vi "SDI-12 Continuous Operations.vi"(0 "RS232 Port In":refnum<visa-resource-name>="COM11", 1 "Sensor Address In":string="0", 3 "Sonde Data Ctl Refnum":refnum<vi>, 4 "Stop Ctl Refnum":refnum<vi>, 5 "Error In (No Error)":errorcluster, 6 "file directory (dialog if empty)":path=path "D:/Cascade/Raw Data files", 7 "Save File":bool) -> (11 "Measurements Out":dbl[](array[numeric]), 12 "new file path (Not A Path if cancelled)":path, 13 "Array":timestamp[](array[timestamp]), 15 "Address Out":string="a" caption="sensor address out", 16 "output cluster":T1 caption="Cluster" {"Dissolved\nOxygen %" format="%_4g"; "Salinity" format="%_3g"; "Temp deg C" format="%_2g"; "ORP" format="%_4g"; "pH" format="%_4g"; "Dissolved\nOxygen mg/L" format="%_4g"; "Specific\nCond (uS)" format="%_4g"}, 17 "Temperature":cluster{"Y":dbl[], "Y":dbl[]}[](graph), 18 "Sonde Data Display":T2, 19 "Error Out":errorcluster)   [LabVIEW 2016]
doc: "A general set of examples of the SDI-12 API for a generic sensor. A tab control separates each example, and contains the following examples:\n1. Read Single.\n2. Read Multiple.\n3. Acknowledge Active.\n4. Change Address.\n5. Address Query.\n6. Send Identification."
uses:
  SDI-12/Sonde Vertical Graph.ctl
  controls/Vertical Chart.ctl
  activeXtest/activeXtest 2015 Folder/sonde cluster.ctl
  <vilib>/Utility/file.llb/Write Delimited Spreadsheet (string).vi
  <vilib>/Utility/file.llb/Write Delimited Spreadsheet (DBL).vi
  SDI-12/SDI-12.lvlib
panel:
  out "Sensor On/Off Response":bool
  out "Battery Voltage (V)":dbl
  out "Number of Measurements Out":i32
  in  "Measurement Type In (Normal)":i32(ring)=1 items=["Normal", "Concurrent", "Continuous"]
  out "Parameter Out":i32(ring) items=["0", "1", "2", "3", "4", "5", "6", "7", "8", "9"]
  in  "Parameter In (0)":i32(ring) items=["0", "1", "2", "3", "4", "5", "6", "7", "8", "9"]
  in  "CRC (False)":bool
  out "CRC Out":bool
  out "Measurement Type Out":i32(ring) items=["Normal", "Concurrent", "Continuous"]
  out "Time (s)":dbl
  in  "stop":bool
  out "counter":i32
  out "start time":timestamp
  # "deg C"
  # "pH"
  # "specific conductance"
  # "salinity"
  # "DO % saturation"
  # "DO mg/L"
  # "ORP"
  # "depth"
  # "battery"
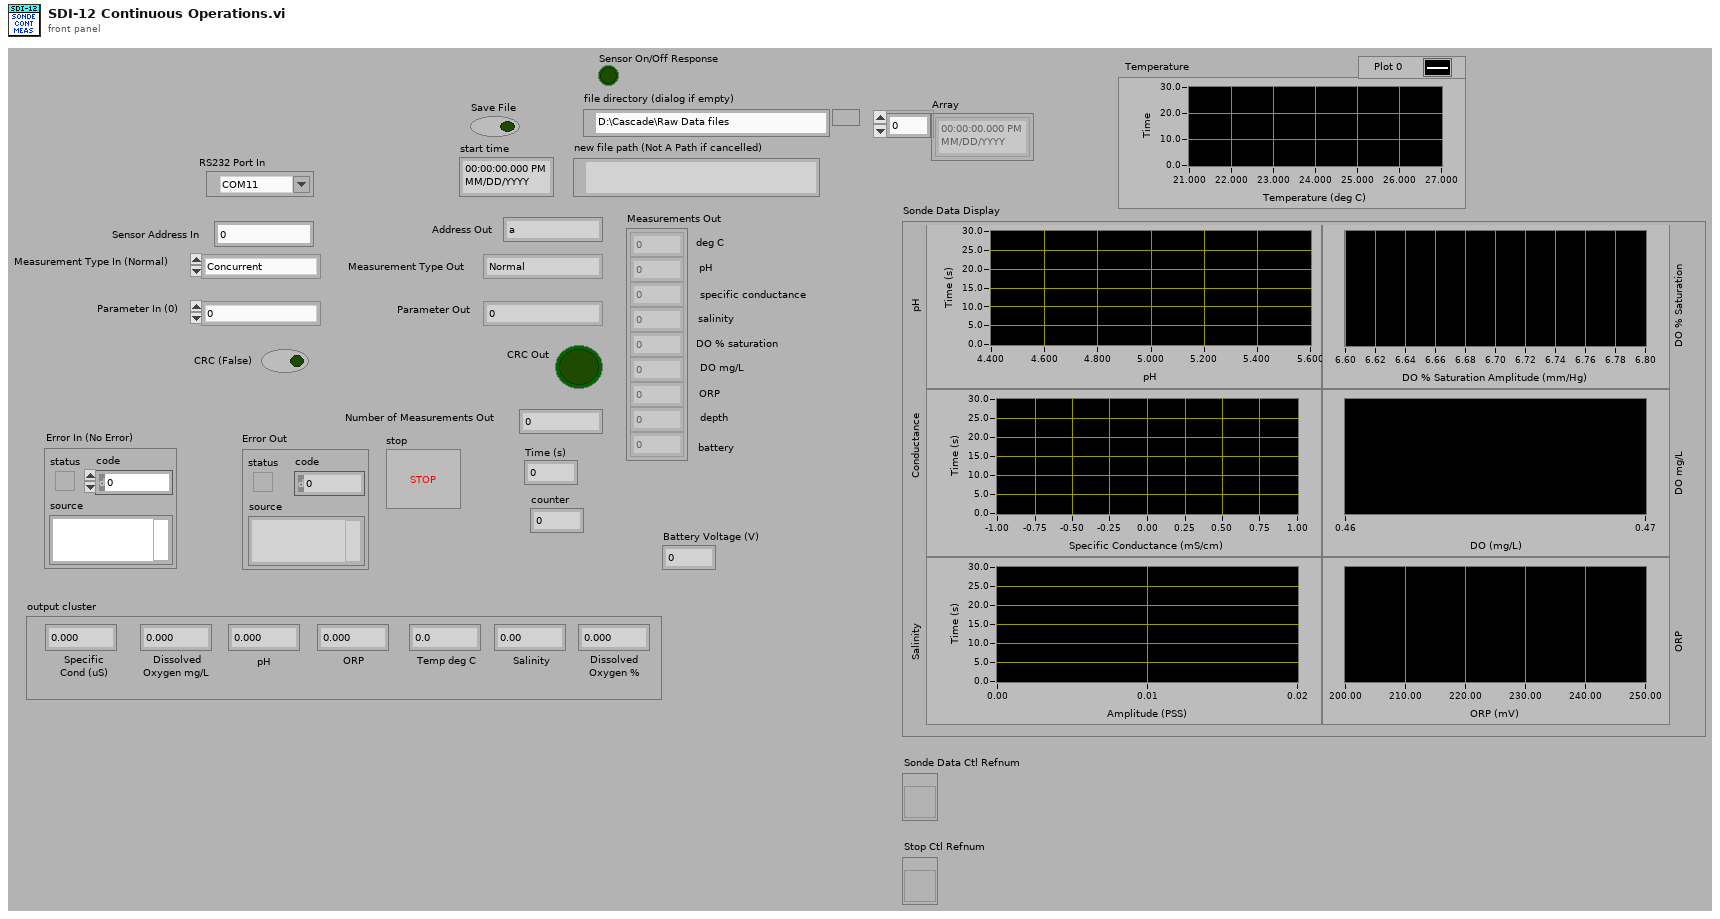
[diagram p1: front panel]
types:
  T1 = typedef "sonde cluster.ctl" = cluster{"Specific\nCond (uS)":dbl, "Dissolved\nOxygen mg/L":dbl, "pH":dbl, "ORP":dbl, "Temp deg C":dbl, "Salinity":dbl, "Dissolved\nOxygen %":dbl}
  T2 = typedef "Sonde Vertical Graph.ctl" = cluster{"pH":T3, "Conductance":T3, "Salinity":T3, "DO % Saturation":T3, "DO mg/L":T3, "ORP":T3}
  T3 = typedef "Vertical Chart.ctl" = cluster{"Y":dbl[], "Y":dbl[]}[]
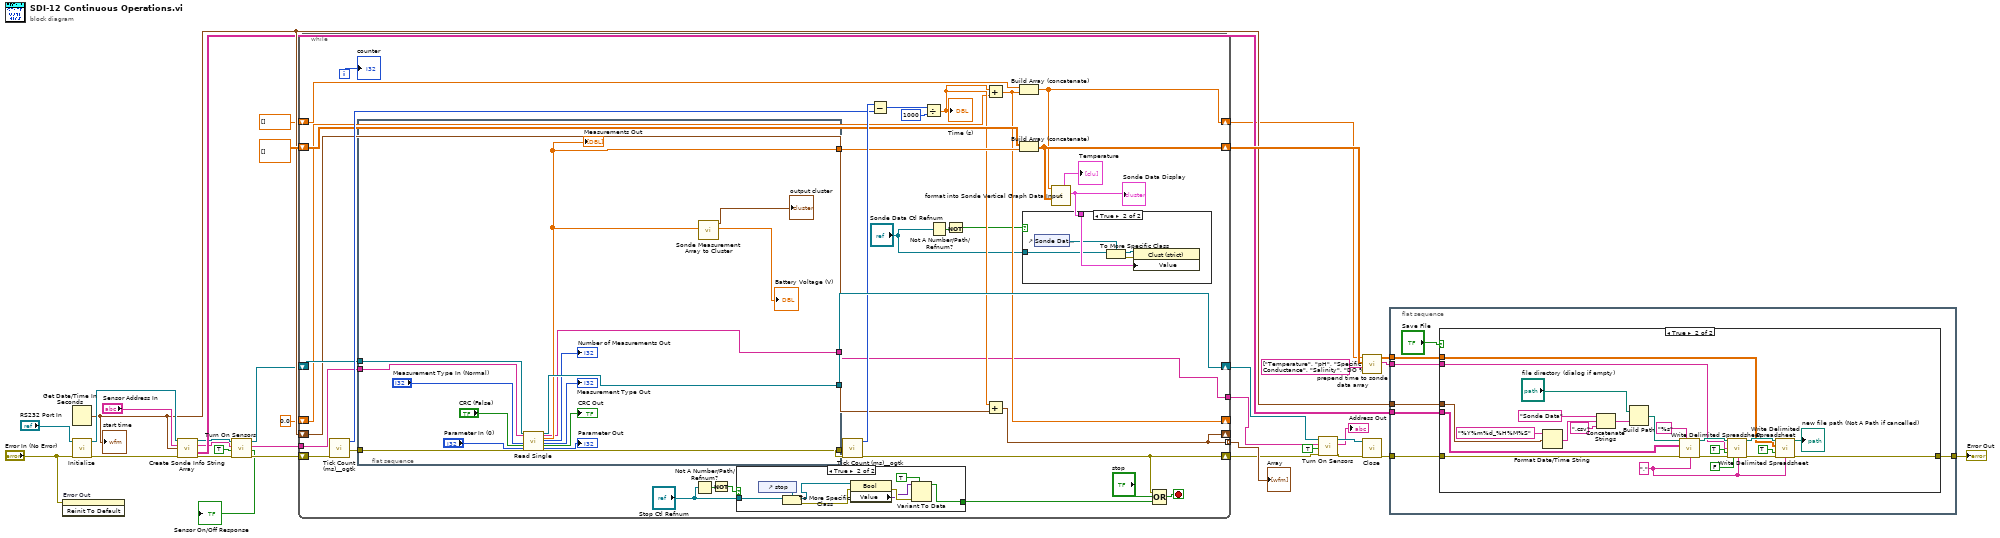
[diagram p0: block diagram]
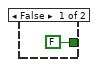
[diagram p3: hidden frame]
diagram:
  n1 = invoke on="Error Out" class="Clust (strict)" method="Reinit To Default"(error in="Error In (No Error)") -> ()  [unwired: 2 in, 3 out]
  n2 = Get Date/Time In Seconds() -> (seconds since 1Jan1904=w23:timestamp)
  "start time" <- w23
  n3 = call "Initialize.vi"("Error In (No Error)"="Error In (No Error)", "RS232 Port In"="RS232 Port In") -> ("Error Out"=w32:errorcluster, "RS232 Port Out"=w31:refnum<visa-resource-name>)  [unwired: 8 in]
  n4 = call "Create Sonde Info String Array.vi"("VISA Refnum in"=w31, "Sensor Address In"="Sensor Address In", "seconds since 1Jan1904"=w23, "error in (no error)"=w32) -> ("VISA Refnum out"=w14:refnum<visa-resource-name>, "Address Out"=w12:string, "Array"=w22:string[][], "error out"=w16:errorcluster)  [unwired: 8 in]
  n5 = call "Turn On Sensors.vi"("Error In (No Error)"=w16, "Sensor On/Off"=TRUE, "Sensor Address In"=w12, "RS232 Port In"=w14) -> ("Error Out"=w15:errorcluster, "Sensor On/Off Response"=→"Sensor On/Off Response":bool, "Address Out"=w11:string, "RS232 Port Out"=w13:refnum<visa-resource-name>)  [unwired: 4 in]
  n6 = while {
    shift-right: [w67] -> w7
    shift-left: w13 -> [w60]
    shift-right: [w43] -> w9
    shift-left: w15 -> [w59]
    shift-right: [w54] -> w28
    shift-left: dbl[][] [] -> [w55]
    tunnel: [w52] -> w29 mode=indexing
    shift-right: [w52] -> _
    shift-left: w23 -> [w53]
    shift-right: [w50] -> w19
    shift-left: dbl[] [] -> [w47]
    tunnel: w11 -> [w51]
    shift-right: [w46] -> _
    shift-left: 0.0 -> [w48]
    tunnel: [w42] -> w5
    i -> [w57]
    stop <- w44 stop-if-true
    n7 = call <userlib>:"Tick Count (ms)__ogtk.vi"("error in (no error)"=w59) -> ("error out"=w65:errorcluster, "millisecond timer value"=w63:u32)  [unwired: 9 in]
    n8 = flat-sequence {
      tunnel: [w97] -> w67
      tunnel: [w96] -> w66
      tunnel: w65 -> [w88]
      tunnel: w60 -> [w87]
      tunnel: [w85] -> w56
      tunnel: w51 -> [w86]
      tunnel: [w84] -> w42
      frame #0 {
        n9 = call "Read Single.vi"("RS232 Port In"=w87, "Sensor Address In"=w86, "Measurement Type In (Normal)"="Measurement Type In (Normal)", "CRC (False)"="CRC (False)", "Parameter In (0)"="Parameter In (0)", "Error In (No Error)"=w88) -> ("RS232 Port Out"=w97:refnum<visa-resource-name>, "Sensor Address Out"=w84:string, "Measurements Out"=w85:dbl[], "Number of Measurements Out"=→"Number of Measurements Out":i32, "Measurement Type Out"=→"Measurement Type Out":i32, "CRC Out"=→"CRC Out":bool, "Parameter Out"=→"Parameter Out":i32, "Error Out"=w96:errorcluster)  [unwired: 14 in]
        "Measurements Out" <- w85
        n10 = call "Sonde Measurement Array to Cluster.vi"("Measurements In"=w85) -> ("Battery Voltage (V)"=→"Battery Voltage (V)":dbl, "Cluster Out"=→"output cluster":T1)  [unwired: 9 in]
      }
    }
    n11 = Not A Number/Path/Refnum?(number/path/refnum="Stop Ctl Refnum") -> (NaN/Path/Refnum?=w37:bool)
    n12 = Not(x=w37) -> (.not. x?=w35:bool)
    n13 = case shown="True" w35 {
      tunnel: "Stop Ctl Refnum" -> [_ w76]
      tunnel: [FALSE w69] -> w34
      frame False {
      }
      frame True {
        n14 = control-ref of="stop"() -> (w74:refnum<vi>)
        n15 = To More Specific Class(target class=w74, reference=w76) -> (specific class reference=w71:refnum<vi>, error out=w75:errorcluster)  [unwired: 1 in]
        n16 = property class="Bool"(reference=w71, error in=w75) -> (error out=w73:errorcluster, "Value"=w72:variant)  [unwired: 1 out]
        n17 = Variant To Data(error in=w73, type=TRUE, Variant=w72) -> (data=w69:bool)  [unwired: 1 out]
      }
    }
    n18 = call <userlib>:"Tick Count (ms)__ogtk.vi"("error in (no error)"=w66) -> ("error out"=w43:errorcluster, "millisecond timer value"=w64:u32)  [unwired: 9 in]
    n19 = Subtract(x=w64, y=w63) -> (x-y=w62:u32)
    n20 = Divide(x=w62, y=u32 1000) -> (x/y=w49:dbl)
    "Time (s)" <- w49
    n21 = Not A Number/Path/Refnum?(number/path/refnum="Sonde Data Ctl Refnum") -> (NaN/Path/Refnum?=w41:bool)
    n22 = Not(x=w41) -> (.not. x?=w40:bool)
    n23 = Add(x=w49, y=w48) -> (x+y=w46:dbl)
    n24 = Add(x=w49, y=w53) -> (x+y=w52:timestamp)
    n25 = Build Array (concatenate)(w47, w46) -> (w50:dbl[])
    n26 = Build Array (concatenate)(w55, w56) -> (w54:dbl[][])
    n27 = call "format into Sonde Vertical Graph Data Input.vi"("Sonde Measurement Array"=w54, "Time Array"=w50) -> ("Sonde Data Display"=w39:T2, "Temperature"=→"Temperature":cluster{"X":dbl[], "Y":dbl[]}[])  [unwired: 8 in]
    "Sonde Data Display" <- w39
    n28 = case shown="True" w40 {
      tunnel: w39 -> [_ w81]
      tunnel: "Sonde Data Ctl Refnum" -> [_ w79]
      frame False {
      }
      frame True {
        n29 = control-ref of="Sonde Data Display"() -> (w80:refnum<vi>)
        n30 = To More Specific Class(target class=w80, reference=w79) -> (specific class reference=w78:refnum<vi>, error out=w77:errorcluster)  [unwired: 1 in]
        n31 = property class="Clust (strict)"(reference=w78, error in=w77, "Value"=w81) -> ()  [unwired: 2 out]
      }
    }
    n32 = Compound Arithmetic op=OR(w43, "stop", w34) -> (w44:bool)
    "counter" <- w57
  }
  "Array" <- w29
  n33 = call "Turn On Sensors.vi"("Error In (No Error)"=w9, "Sensor On/Off"=TRUE, "Sensor Address In"=w5, "RS232 Port In"=w7) -> ("Error Out"=w8:errorcluster, "Address Out"=→"Address Out":string, "RS232 Port Out"=w6:refnum<visa-resource-name>)  [unwired: 4 in, 1 out]
  n34 = call "prepend time to sonde data array.vi"("Measurement Labels"=string[] ["Temperature", "pH", "Specific Conductance", "Salinity", "DO % saturation", "DO", "ORP", "depth", "battery"], "Sonde\nData Array"=w28, "Time Array"=w19) -> ("Header Array"=w21:string[], "Data Array"=w25:dbl[][])  [unwired: 7 in]
  n35 = call "Close.vi"("Error In (No Error)"=w8, "RS232 Port In"=w6) -> ("Error Out"=w27:errorcluster)  [unwired: 9 in]
  n36 = flat-sequence {
    tunnel: w27 -> [w104]
    tunnel: [w103] -> w26
    tunnel: w21 -> [w101]
    tunnel: w25 -> [w100]
    tunnel: w23 -> [w99]
    tunnel: w22 -> [w98]
    frame #0 {
      n37 = case shown="True" "Save File" {
        tunnel: [w105 w125] -> w103
        tunnel: w104 -> [w105 w110]
        tunnel: w101 -> [_ w106]
        tunnel: w100 -> [_ w123]
        tunnel: w99 -> [_ w117]
        tunnel: w98 -> [_ w108]
        frame False {
        }
        frame True {
          w107 = "," ("delimiter (\\t)")
          n38 = Format Date/Time String(time format string (%c)="%Y%m%d_%H%M%S", seconds (now)=w117) -> (date/time string=w116:string)  [unwired: 1 in]
          n39 = Concatenate Strings("Sonde Data" ("name or relative path"), w116, ".csv" ("string")) -> (w118:string)
          n40 = Build Path(base path="file directory (dialog if empty)", name or relative path=w118) -> (appended path=w113:path)
          n41 = call-poly <vilib>:"Write Delimited Spreadsheet.vi"("file path (dialog if empty)"=w113, "format (%s)"="%s" ("format (%.3f)"), "2D data"=w108, "error in (no error)"=w110, "delimiter (\\t)"=w107) -> ("new file path (Not A Path if cancelled)"=w112:path, "error out"=w109:errorcluster)  [unwired: 9 in]
          n42 = call-poly <vilib>:"Write Delimited Spreadsheet.vi"("file path (dialog if empty)"=w112, "1D data"=w106, "append to file? (new file:F)"=TRUE ("append to file? (F)"), "error in (no error)"=w109, "transpose? (no:F)"=FALSE ("transpose? (F)"), "delimiter (\\t)"=w107) -> ("new file path (Not A Path if cancelled)"=w127:path, "error out"=w126:errorcluster)  [unwired: 8 in]
          n43 = call-poly <vilib>:"Write Delimited Spreadsheet.vi"("file path (dialog if empty)"=w127, "2D data"=w123, "append to file? (new file:F)"=TRUE ("append to file? (F)"), "error in (no error)"=w126, "delimiter (\\t)"=w107) -> ("new file path (Not A Path if cancelled)"=→"new file path (Not A Path if cancelled)":path, "error out"=w125:errorcluster)  [unwired: 9 in]
        }
      }
    }
  }
  "Error Out" <- w26
